vi "Find Nearest Edge.vi"(7 "Pane Coordinates":T3, 8 "error in (no error)":errorcluster, 11 "Boolean Object Position in":refnum<class "Boolean Object Position.lvclass">) -> (0 "error out":errorcluster, 1 "Direction":T1, 2 "Nearest Side":T2=enum."Top", 3 "Boolean Object Position out":refnum<class "Boolean Object Position.lvclass">)   [LabVIEW 2018, in "Boolean Object Position.lvclass"]
uses:
  Boolean Object Position.lvclass
  Pane Object.lvclass/Object Coordinates.ctl
  Pane Object.lvclass/Pane Position Enum.ctl
  Pane Object.lvclass/Direction Ctl.ctl
  Pane Object.lvclass/Pane Object Position.lvclass
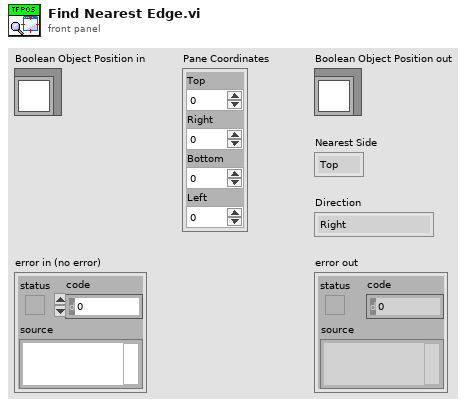
[diagram p1: front panel]
types:
  T1 = typedef "Direction Ctl.ctl" = enum16{"Right", "Left", "Up", "Down"}
  T2 = typedef "Pane Object Position.lvclass/Pane Position Enum.ctl" = enum16{"Indeterminate", "Top", "Right", "Top Right", "Bottom", "5", "Bottom Right", "7", "Left", "Top Left", "10", "11", "Bottom Left"}
  T3 = typedef "Pane Object Position.lvclass/Object Coordinates.ctl" = cluster{"Top":i32, "Right":i32, "Bottom":i32, "Left":i32}
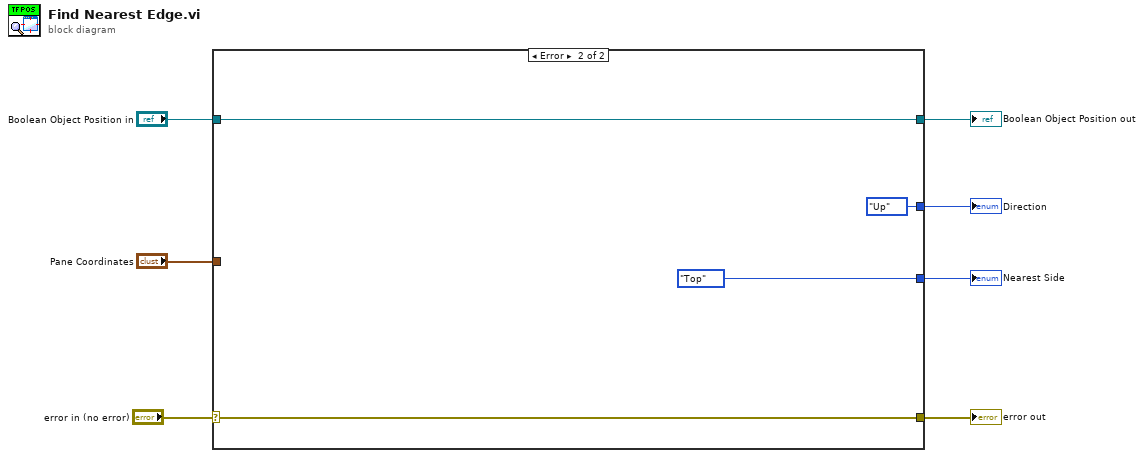
[diagram p0: block diagram]
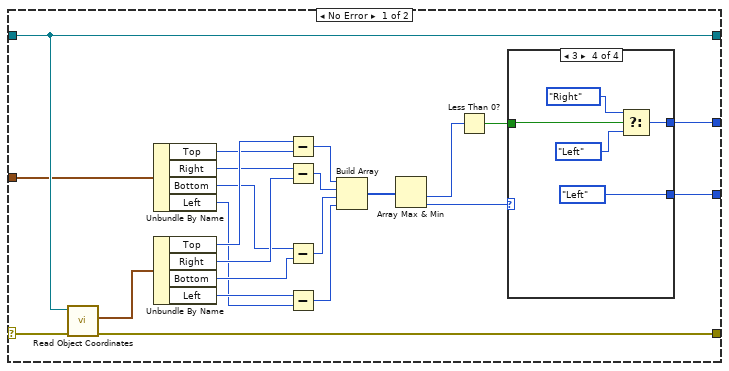
[diagram p2: hidden frame]
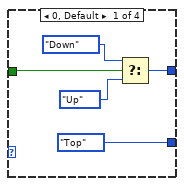
[diagram p3: hidden frame]
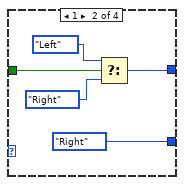
[diagram p4: hidden frame]
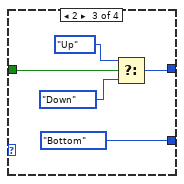
[diagram p5: hidden frame]
diagram:
  n1 = case shown="Error" "error in (no error)" {
    selector: "error in (no error)" -> [w29 w54]
    tunnel: [w28 w54] -> w6
    tunnel: "Boolean Object Position in" -> [w30 w53]
    tunnel: [w30 w53] -> w4
    tunnel: "Pane Coordinates" -> [w27 _]
    tunnel: [w11 Pane_Position_Enum."Top" ("Nearest Side")] -> w2
    tunnel: [w8 Direction_Ctl."Up" ("Direction")] -> w1
    frame No Error {
      n2 = call-dynamic "Read Object Coordinates.vi"("error in (no error)"=w29, "Pane Object Position in"=w30) -> ("error out"=w28:errorcluster, "Object Coordinates"=w26:T3)  [unwired: 7 in, 1 out]
      n3 = Unbundle By Name(w27) -> ("Top"=w24:i32, "Right"=w22:i32, "Bottom"=w21:i32, "Left"=w18:i32)
      n4 = Unbundle By Name(w26) -> ("Top"=w25:i32, "Right"=w23:i32, "Bottom"=w20:i32, "Left"=w19:i32)
      n5 = Subtract(x=w25, y=w24) -> (x-y=w17:i32)
      n6 = Subtract(x=w22, y=w23) -> (x-y=w16:i32)
      n7 = Subtract(x=w21, y=w20) -> (x-y=w15:i32)
      n8 = Subtract(x=w19, y=w18) -> (x-y=w14:i32)
      n9 = Build Array(w17, w16, w15, w14) -> (w13:i32[])
      n10 = Array Max & Min(array=w13) -> (min value=w10:i32, min index (indices)=w12:i32)  [unwired: 2 out]
      n11 = Less Than 0?(x=w10) -> (x < 0?=w9:bool)
      n12 = case shown="3" w12 {
        tunnel: [Pane_Position_Enum."Top" ("Nearest Side") Pane_Position_Enum."Right" ("Nearest Side") Pane_Position_Enum."Bottom" ("Nearest Side") Pane_Position_Enum."Left" ("Nearest Side")] -> w11
        tunnel: w9 -> [w31 w39 w41 w46]
        tunnel: [w32 w36 w42 w47] -> w8
        frame 0, Default {
          n13 = Select(t=Direction_Ctl."Down" ("Direction"), s=w31, f=Direction_Ctl."Up" ("Direction")) -> (s? t:f=w32:T1)
        }
        frame 1 {
          n14 = Select(t=Direction_Ctl."Left" ("Direction"), s=w39, f=Direction_Ctl."Right" ("Direction")) -> (s? t:f=w36:T1)
        }
        frame 2 {
          n15 = Select(t=Direction_Ctl."Up" ("Direction"), s=w41, f=Direction_Ctl."Down" ("Direction")) -> (s? t:f=w42:T1)
        }
        frame 3 {
          n16 = Select(t=Direction_Ctl."Right" ("Direction"), s=w46, f=Direction_Ctl."Left" ("Direction")) -> (s? t:f=w47:T1)
        }
      }
    }
    frame Error {
    }
  }
  "error out" <- w6
  "Boolean Object Position out" <- w4
  "Nearest Side" <- w2
  "Direction" <- w1
